vi "Controller Load Configuration.vi"(8 "error in (no error)":errorcluster) -> (0 "error out":errorcluster, 3 "FOFB Configuration":T1={"FOFB Parameters"={"Network"={"FOFB Controller IP"="", "LNLS Control Network IP"="", "LNLS Control Network Power Supplies TCP Port"=0, "LNLS Control Network FOFB Configuration TCP Port"=0, "Data Server TCP Port"=0, "Monitoring Data TCP Port"=0, "Configuration GUI TCP Port"=0, "TCP Listening Timeout"=0}, "Fast Acquisition"={"Acquisition Period"=0, "Data Buffer Size"=0}, "Response Matrix Measurement"={"Step Amplitude"=0.0, "Time Between Steps"=0, "Step Duration"=0, "Number of Averages"=0}, "Correction Algorithm"={"Correction Period"=0, "Reference Orbit Path"=path "", "Response Matrix Path"=path "", "Correction Matrix Path"=path "", "Horizontal Correction Factor"=0.0, "Vertical Correction Factor"=0.0, "Beam Current FOFB Threshold"=0.0, "Decouple H-V"=FALSE}, "Acquisition Network"=[], "Actuation Network"=[]}, "Number of Acquisition Chassis"=0, "Number of Actuation Chassis"=0, "Number of BPM Readings"=0, "BPM Reading Names"=[], "Selected BPM Readings"=[0, 1, 2, 3, 4, 5, 6, 7, 8, 9, 10, 11, 12, 13, 14, 15, 16, 17, 18, 19, 20, 21, 22, 23, 24, 25, 26, 27, 28, 29, 30, 31, 32, 33, 34, 35, 36, 37, 38, 39, 40, 41, 42, 43, 44, 45, 46, 47, 48, 49], "Number of Correctors"=0, "Corrector Names"=[], "Selected Correctors"=[0, 1, 2, 3, 4, 5, 6, 7, 8, 9, 10, 11, 12, 13, 14, 15, 16, 17, 18, 19, 20, 21, 22, 23, 24, 25, 26, 27, 28, 29, 30, 31, 32, 33, 34, 35, 36, 37, 38, 39, 40, 41, 42, 43, 44, 45, 46, 47, 48, 49], "Reference Orbit"=[], "Response Matrix"=[], "Correction Matrix"=[], "Acquisition Chassis Names"=[], "Actuation Chassis Names"=[], "Acquisition Variables"=[], "Actuation Variables"=[], "PS Matrix Mapping"=[], "Inverse PS Matrix Mapping"=[], "Response Matrix Beam Energy (MeV)"=0.0, "PID Parameters"=[], "BPM Planes"=[], "Corrector Planes"=[], "RMM Step Factor"=[]})   [LabVIEW 2011, in "Controller VIs.lvlib"]
doc: "Load the FOFB Controller configuration and parameters from a configuration file and builds the configuration cluster (FOFB Configuration) used thorough the program execution. Perform tasks related with the FOFB configuration, such as change of Scan Engine period, load response matrix from file, load reference orbit from file, calculate correction matrix."
uses:
  Controller VIs.lvlib
  Types Definitions/Type FOFB Configuration.ctl
  Types Definitions/Type FOFB Parameters.ctl
  Types Definitions/Type Network Configuration.ctl
  Types Definitions/Type FA Configuration.ctl
  Types Definitions/Type Response Matrix Measurement Configuration.ctl
  Types Definitions/Type Correction Algorithm Configuration.ctl
  Types Definitions/Type Acquisition Network Configuration.ctl
  Types Definitions/Type Actuation Network Configuration.ctl
  Types Definitions/Type PID Parameters.ctl
  XML VIs.lvlib
  Type Definitions.lvlib
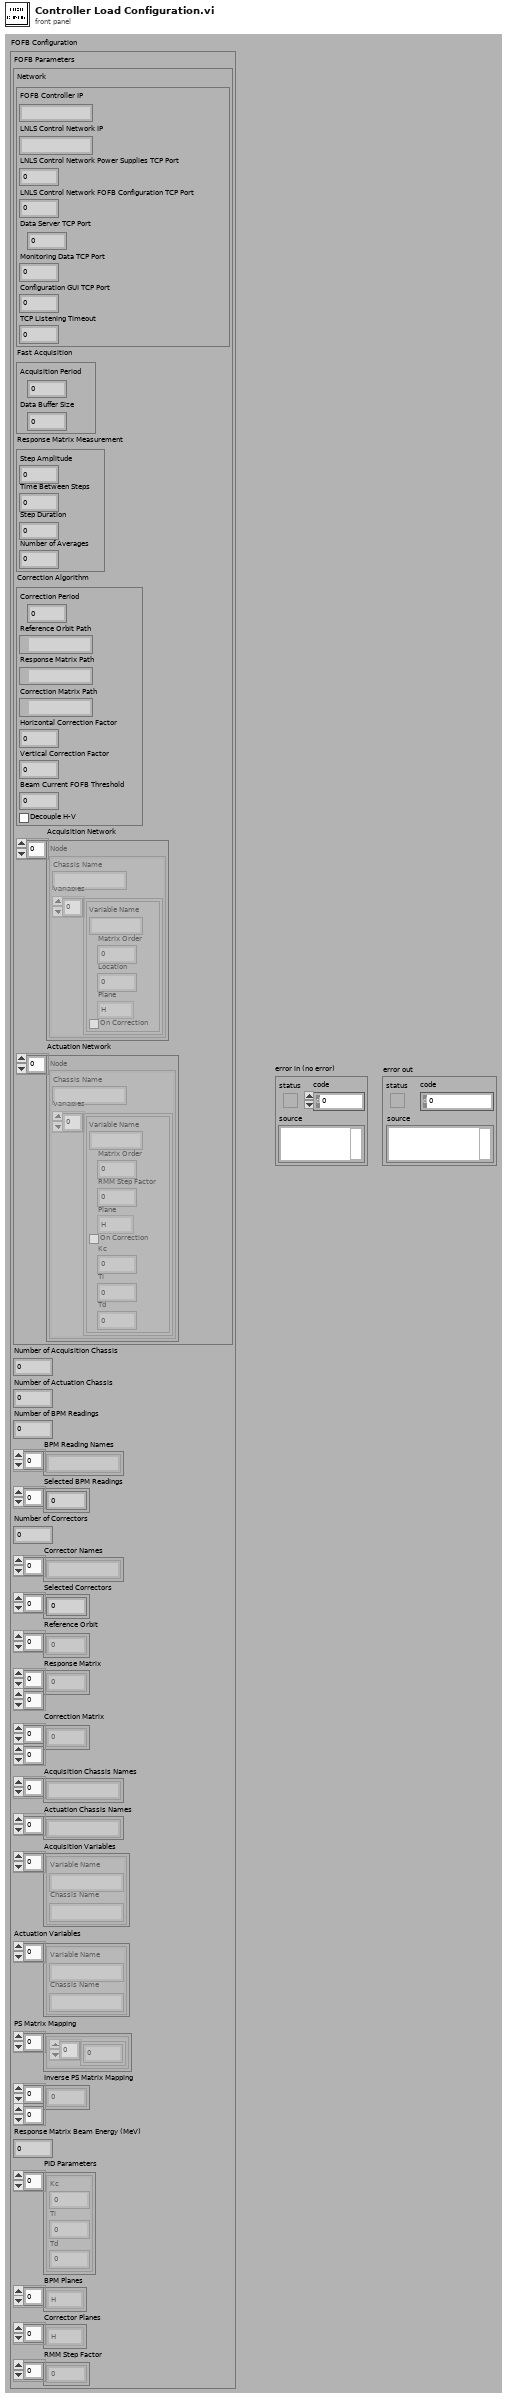
[diagram p1: front panel]
types:
  T1 = typedef "Type Definitions.lvlib/Type FOFB Configuration.ctl" = cluster{"FOFB Parameters":T2, "Number of Acquisition Chassis":i32, "Number of Actuation Chassis":i32, "Number of BPM Readings":i32, "BPM Reading Names":string[], "Selected BPM Readings":u32[], "Number of Correctors":i32, "Corrector Names":string[], "Selected Correctors":u32[], "Reference Orbit":dbl[], "Response Matrix":dbl[][], "Correction Matrix":dbl[][], "Acquisition Chassis Names":string[], "Actuation Chassis Names":string[], "Acquisition Variables":cluster{"Variable Name":string, "Chassis Name":string}[], "Actuation Variables":cluster{"Variable Name":string, "Chassis Name":string}[], "PS Matrix Mapping":cluster{u32[]}[], "Inverse PS Matrix Mapping":u32[][], "Response Matrix Beam Energy (MeV)":dbl, "PID Parameters":T9[], "BPM Planes":enum8{"H", "V"}[], "Corrector Planes":enum8{"H", "V"}[], "RMM Step Factor":dbl[]}
  T2 = typedef "Type Definitions.lvlib/Type FOFB Parameters.ctl" = cluster{"Network":T3, "Fast Acquisition":T4, "Response Matrix Measurement":T5, "Correction Algorithm":T6, "Acquisition Network":T7, "Actuation Network":T8}
  T3 = typedef "Type Definitions.lvlib/Type Network Configuration.ctl" = cluster{"FOFB Controller IP":string, "LNLS Control Network IP":string, "LNLS Control Network Power Supplies TCP Port":u16, "LNLS Control Network FOFB Configuration TCP Port":u16, "Data Server TCP Port":u16, "Monitoring Data TCP Port":u16, "Configuration GUI TCP Port":u16, "TCP Listening Timeout":i32}
  T4 = typedef "Type Definitions.lvlib/Type FA Configuration.ctl" = cluster{"Acquisition Period":u32, "Data Buffer Size":u32}
  T5 = typedef "Type Definitions.lvlib/Type Response Matrix Measurement Configuration.ctl" = cluster{"Step Amplitude":dbl, "Time Between Steps":u32, "Step Duration":u32, "Number of Averages":u32}
  T6 = typedef "Type Definitions.lvlib/Type Correction Algorithm Configuration.ctl" = cluster{"Correction Period":u32, "Reference Orbit Path":path, "Response Matrix Path":path, "Correction Matrix Path":path, "Horizontal Correction Factor":dbl, "Vertical Correction Factor":dbl, "Beam Current FOFB Threshold":dbl, "Decouple H-V":bool}
  T7 = typedef "Type Definitions.lvlib/Type Acquisition Network Configuration.ctl" = cluster{"Chassis Name":string, "Variables":cluster{"Variable Name":string, "Matrix Order":u32, "Location":dbl, "Plane":enum8{"H", "V"}, "On Correction":bool}[]}[]
  T8 = typedef "Type Definitions.lvlib/Type Actuation Network Configuration.ctl" = cluster{"Chassis Name":string, "Variables":cluster{"Variable Name":string, "Matrix Order":u32, "RMM Step Factor":dbl, "Plane":enum8{"H", "V"}, "On Correction":bool, "Kc":dbl, "Ti":dbl, "Td":dbl}[]}[]
  T9 = typedef "Type Definitions.lvlib/Type PID Parameters.ctl" = cluster{"Kc":fxp<+/-,16,8>, "Ti":fxp<+/-,16,8>, "Td":fxp<+/-,16,8>}
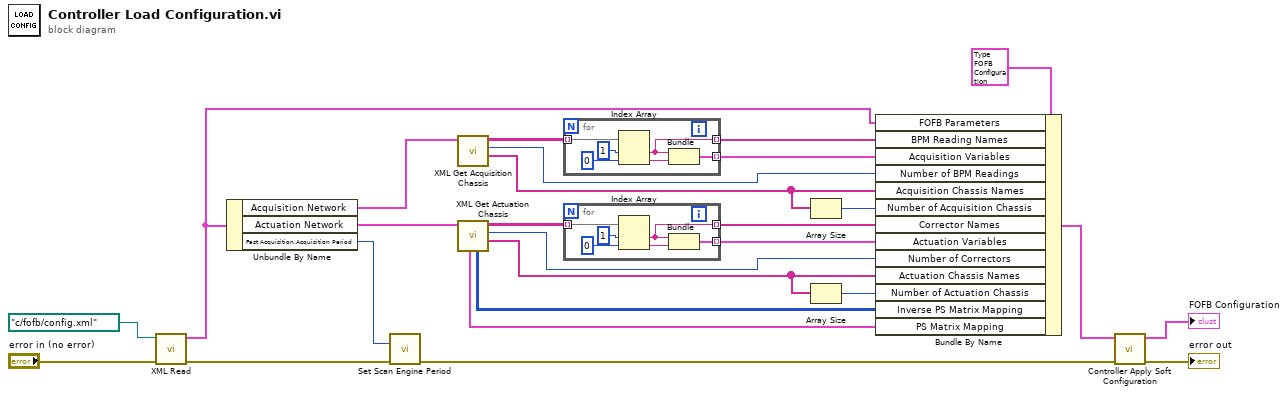
[diagram p0: block diagram]
diagram:
  n1 = call "XML Read.vi"("error in"="error in (no error)", "XML File Path In"=path "c:/fofb/config.xml" ("Configuration File Path")) -> ("error out"=w16:errorcluster, "FOFB Parameters"=w4:T2)  [unwired: 8 in]
  n2 = Unbundle By Name(w4) -> ("Acquisition Network"=w23:T7, "Actuation Network"=w9:T8, "Fast Acquisition.Acquisition Period"=w12:u32)
  n3 = call <vilib>:"Set Scan Engine Period.vi"("scan period (uSec)"=w12, "error in (no error)"=w16) -> ("error out"=w15:errorcluster)  [unwired: 13 in]
  n4 = call "XML Get Acquisition Chassis.vi"("Acquisition Network"=w23) -> ("Acquisition Chassis Names"=w10:string[], "Number of BPM Readings"=w3:i32, "Acquisition Variable Names"=w8:string[][])  [unwired: 4 in, 4 out]
  n5 = call "XML Get Actuation Chassis.vi"("Actuation Network"=w9) -> ("Actuation Chassis Names"=w19:string[], "Number of Correctors"=w5:i32, "Actuation Variable Names"=w21:string[][], "Inverse PS Matrix Mapping"=w18:u32[][], "PS Matrix Mapping"=w1:cluster{u32[]}[])  [unwired: 3 in, 3 out]
  n6 = for {
    tunnel: w8 -> [w31] mode=indexing
    tunnel: [w30] -> w6 mode=indexing
    tunnel: [w27] -> w7 mode=indexing
    n7 = Index Array(array=w31, index #1=1 ("index"), index #2=0 ("index")) -> (element #1=w27:string, element #2=w29:string)
    n8 = Bundle(w27, w29) -> (w30:cluster{string, string})  [unwired: 1 in]
  }
  n9 = for {
    tunnel: w21 -> [w37] mode=indexing
    tunnel: [w36] -> w20 mode=indexing
    tunnel: [w33] -> w11 mode=indexing
    n10 = Index Array(array=w37, index #1=1 ("index"), index #2=0 ("index")) -> (element #1=w33:string, element #2=w35:string)
    n11 = Bundle(w33, w35) -> (w36:cluster{string, string})  [unwired: 1 in]
  }
  n12 = Array Size(array=w10) -> (size(s)=w22:i32)
  n13 = Array Size(array=w19) -> (size(s)=w2:i32)
  n14 = Bundle By Name(cluster=T1 {"FOFB Parameters"={"Network"={"FOFB Controller IP"="", "LNLS Control Network IP"="", "LNLS Control Network Power Supplies TCP Port"=0, "LNLS Control Network FOFB Configuration TCP Port"=0, "Data Server TCP Port"=0, "Monitoring Data TCP Port"=0, "Configuration GUI TCP Port"=0, "TCP Listening Timeout"=0}, "Fast Acquisition"={"Acquisition Period"=0, "Data Buffer Size"=0}, "Response Matrix Measurement"={"Step Amplitude"=0.0, "Time Between Steps"=0, "Step Duration"=0, "Number of Averages"=0}, "Correction Algorithm"={"Correction Period"=0, "Reference Orbit Path"=path "", "Response Matrix Path"=path "", "Correction Matrix Path"=path "", "Horizontal Correction Factor"=0.0, "Vertical Correction Factor"=0.0, "Beam Current FOFB Threshold"=0.0, "Decouple H-V"=FALSE}, "Acquisition Network"=[], "Actuation Network"=[]}, "Number of Acquisition Chassis"=0, "Number of Actuation Chassis"=0, "Number of BPM Readings"=0, "BPM Reading Names"=[], "Selected BPM Readings"=[], "Number of Correctors"=0, "Corrector Names"=[], "Selected Correctors"=[], "Reference Orbit"=[], "Response Matrix"=[], "Correction Matrix"=[], "Acquisition Chassis Names"=[], "Actuation Chassis Names"=[], "Acquisition Variables"=[], "Actuation Variables"=[], "PS Matrix Mapping"=[], "Inverse PS Matrix Mapping"=[], "Response Matrix Beam Energy (MeV)"=0.0, "PID Parameters"=[], "BPM Planes"=[], "Corrector Planes"=[], "RMM Step Factor"=[]}, "FOFB Parameters"=w4, "BPM Reading Names"=w7, "Acquisition Variables"=w6, "Number of BPM Readings"=w3, "Acquisition Chassis Names"=w10, "Number of Acquisition Chassis"=w22, "Corrector Names"=w11, "Actuation Variables"=w20, "Number of Correctors"=w5, "Actuation Chassis Names"=w19, "Number of Actuation Chassis"=w2, "Inverse PS Matrix Mapping"=w18, "PS Matrix Mapping"=w1) -> (w13:T1)
  n15 = call "Controller Apply Soft Configuration.vi"("error in (no error)"=w15, "FOFB Configuration"=w13) -> ("error out"=→"error out":errorcluster, "FOFB Configuration"=→"FOFB Configuration":T1)  [unwired: 8 in]
